vi "get.vi"(10 "variables":string[](array[string])=["intout", "stringout", "time"], 11 "Experience ID":string="Test") -> (0 "error out":errorcluster={"status"=TRUE, "code"=1, "source"="Entry not found"}, 2 "values":string[](array[string])=["0"], 3 "names":string[](array[string])=["intout"])   [LabVIEW 2015]
panel:
  # "Get"
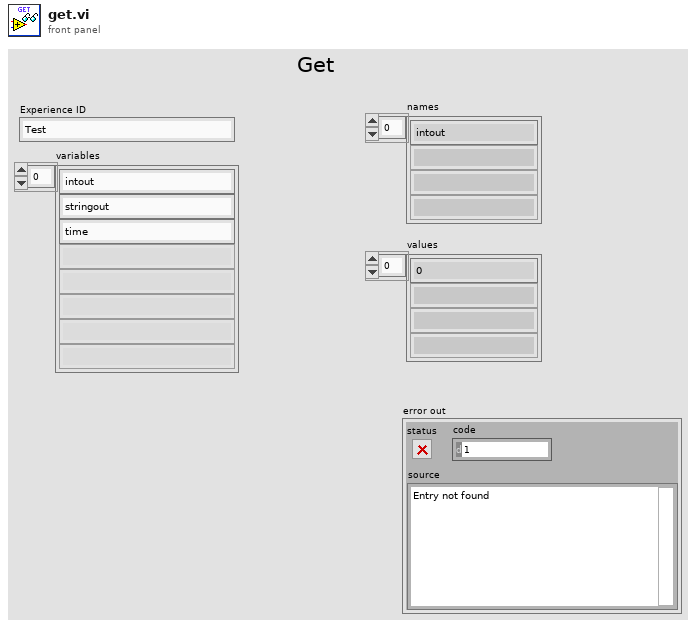
[diagram p1: front panel]
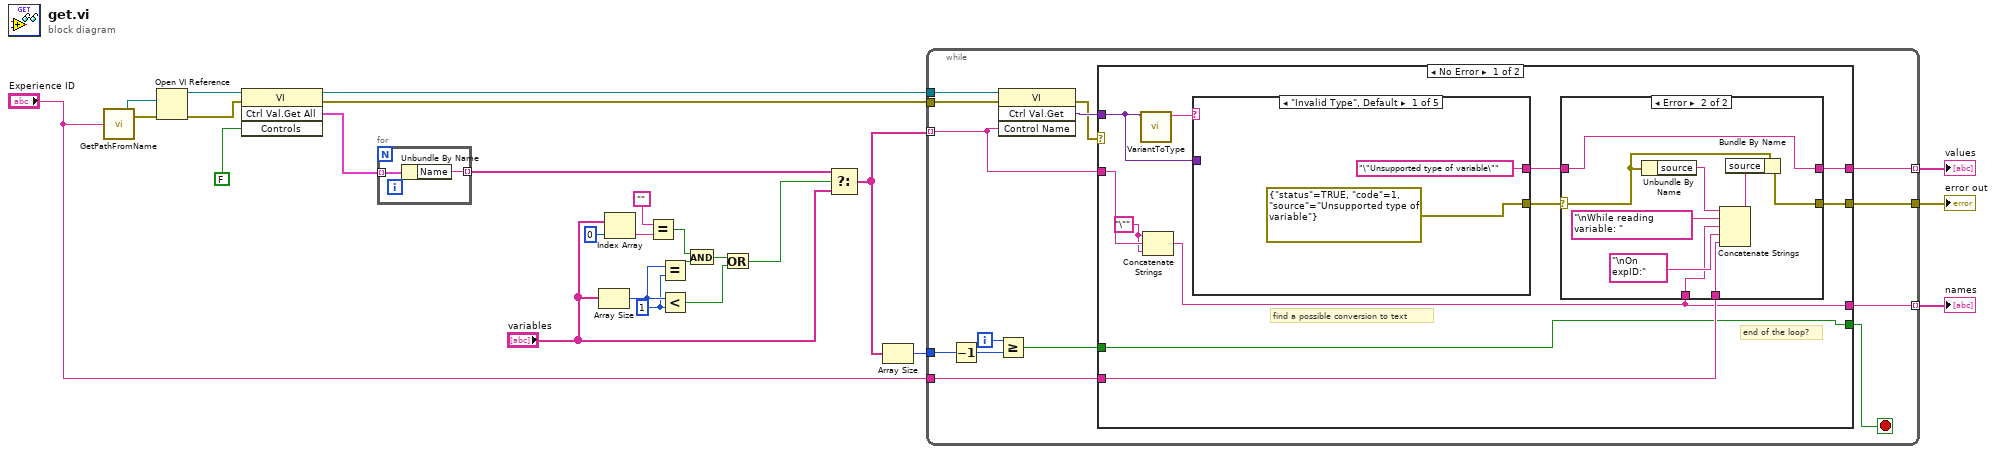
[diagram p0: block diagram]
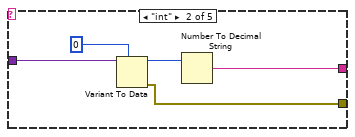
[diagram p3: hidden frame]
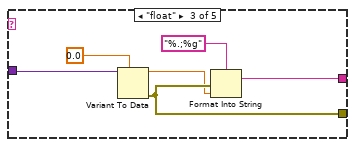
[diagram p4: hidden frame]
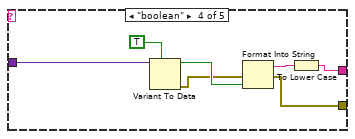
[diagram p5: hidden frame]
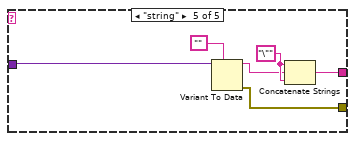
[diagram p6: hidden frame]
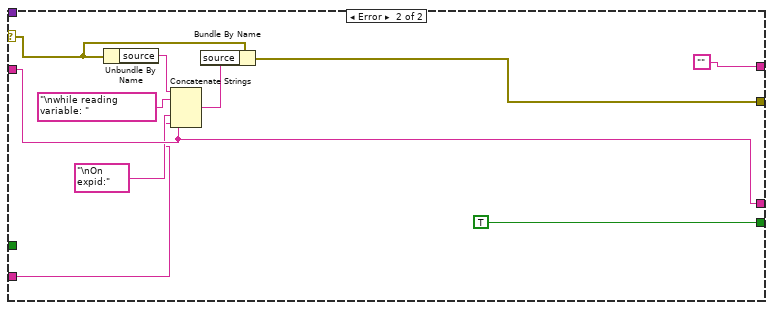
[diagram p7: hidden frame]
diagram:
  w11 = 1 ("y")
  n1 = call "GetPathFromName.vi"("Experience ID"="Experience ID") -> ("Error out"=w25:errorcluster, "VI_Path"=w26:path)
  n2 = Open VI Reference(vi path=w26, error in (no error)=w25) -> (vi reference=w19:refnum<vi>, error out=w8:errorcluster)  [unwired: 1 in, 3 out]
  n3 = invoke class="VI" method="Ctrl Val.Get All"(reference=w19, error in=w8, "Controls"=FALSE) -> (reference out=w18:refnum<vi>, error out=w7:errorcluster, "Get All Control Values Variant"=w16:cluster{"Name":string, "Variant Data":variant}[])  [unwired: 1 in, 1 out]
  n4 = for {
    tunnel: w16 -> [w28] mode=indexing
    tunnel: [w27] -> w15 mode=indexing
    n5 = Unbundle By Name(w28) -> ("Name"=w27:string)
  }
  n6 = Array Size(array="variables") -> (size(s)=w12:i32)
  n7 = Index Array(array="variables", index=0) -> (element=w2:string)
  n8 = Equal?(x="", y=w2) -> (x = y?=w5:bool)
  n9 = Equal?(x=w12, y=w11) -> (x = y?=w9:bool)
  n10 = Less?(x=w12, y=w11) -> (x < y?=w13:bool)
  n11 = And(x=w5, y=w9) -> (x .and. y?=w10:bool)
  n12 = Or(x=w10, y=w13) -> (x .or. y?=w1:bool)
  n13 = Select(t=w15, s=w1, f="variables") -> (s? t:f=w14:string[])
  n14 = Array Size(array=w14) -> (size(s)=w24:i32)
  n15 = while {
    tunnel: w14 -> [w37] mode=indexing
    tunnel: w18 -> [w42]
    tunnel: w24 -> [w32]
    tunnel: w7 -> [w41]
    tunnel: [w36] -> w20
    tunnel: [w35] -> w23 mode=indexing
    tunnel: [w34] -> w22 mode=indexing
    tunnel: "Experience ID" -> [w33]
    i -> [w30]
    stop <- w38 stop-if-true
    n16 = Decrement(x=w32) -> (x-1=w29:i32)
    n17 = Greater Or Equal?(x=w30, y=w29) -> (x >= y?=w31:bool)
    n18 = invoke class="VI" method="Ctrl Val.Get"(reference=w42, error in=w41, "Control Name"=w37) -> (error out=w39:errorcluster, "Get Control Value Variant"=w40:variant)  [unwired: 1 in, 2 out]
    n19 = case shown="No Error" w39 {
      selector: w39 -> [_ w99]
      tunnel: w40 -> [w45 _]
      tunnel: w31 -> [w43 _]
      tunnel: [w43 TRUE] -> w38
      tunnel: w37 -> [w47 w94]
      tunnel: [w52 w95] -> w36
      tunnel: [w50 ""] -> w35
      tunnel: [w48 w94] -> w34
      tunnel: w33 -> [w49 w91]
      frame No Error {
        w46 = "\"" ("string")
        # "end of the loop?"
        # "find a possible conversion to text"
        n20 = call "VariantToType.vi"("Variant"=w45) -> ("type Name"=w44:string)  [unwired: 10 in]
        n21 = Concatenate Strings(w46, w47, w46) -> (w48:string)
        n22 = case shown="\"Invalid Type\", Default" w44 {
          tunnel: w45 -> [_ w70 w76 w82 w89]
          tunnel: ["\"Unsupported type of variable\"" w68 w72 w78 w85] -> w51
          tunnel: [errorcluster {"status"=TRUE, "code"=1, "source"="Unsupported type of variable"} ("error out") w67 w75 w80 w88] -> w53
          frame "Invalid Type", Default {
          }
          frame "int" {
            n23 = Variant To Data(type=0, Variant=w70) -> (data=w69:i32, error out=w67:errorcluster)  [unwired: 1 in]
            n24 = Number To Decimal String(number=w69) -> (decimal integer string=w68:string)  [unwired: 1 in]
          }
          frame "float" {
            n25 = Variant To Data(type=0.0, Variant=w76) -> (data=w74:dbl, error out=w75:errorcluster)  [unwired: 1 in]
            n26 = Format Into String(format string="%.;%g", error in=w75, w74) -> (resulting string=w72:string)  [unwired: 1 in, 1 out]
          }
          frame "boolean" {
            n27 = Variant To Data(type=TRUE, Variant=w82) -> (data=w84:bool, error out=w83:errorcluster)  [unwired: 1 in]
            n28 = Format Into String(error in=w83, w84) -> (resulting string=w79:string, error out=w80:errorcluster)  [unwired: 2 in]
            n29 = To Lower Case(string=w79) -> (all lower case string=w78:string)
          }
          frame "string" {
            w87 = "\"" ("string")
            n30 = Variant To Data(type="", Variant=w89) -> (data=w86:string, error out=w88:errorcluster)  [unwired: 1 in]
            n31 = Concatenate Strings(w87, w86, w87) -> (w85:string)
          }
        }
        n32 = case shown="Error" w53 {
          selector: w53 -> [w55 w63]
          tunnel: [w55 w64] -> w52
          tunnel: [w54 w56] -> w50
          tunnel: w51 -> [w54 w56]
          tunnel: w48 -> [_ w58]
          tunnel: w49 -> [_ w57]
          frame No Error {
            # "add to the list"
          }
          frame Error {
            n33 = Unbundle By Name(w63) -> ("source"=w62:string)
            n34 = Concatenate Strings(w62, "\nWhile reading variable: " ("string"), w58, "\nOn expID:" ("string"), w57) -> (w60:string)
            n35 = Bundle By Name(cluster=w63, "source"=w60) -> (w64:errorcluster)
          }
        }
      }
      frame Error {
        n36 = Unbundle By Name(w99) -> ("source"=w98:string)
        n37 = Concatenate Strings(w98, "\nwhile reading variable: " ("string"), w94, "\nOn expid:", w91) -> (w96:string)
        n38 = Bundle By Name(cluster=w99, "source"=w96) -> (w95:errorcluster)
      }
    }
  }
  "error out" <- w20
  "names" <- w22
  "values" <- w23
